vi "mathforthing.vi"(9 "setpoint":dbl, 10 "starting angle":dbl) -> (2 "output":dbl)   [LabVIEW 2020]
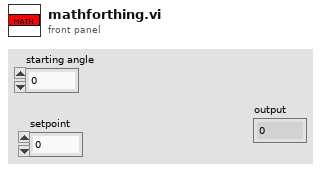
[diagram p1: front panel]
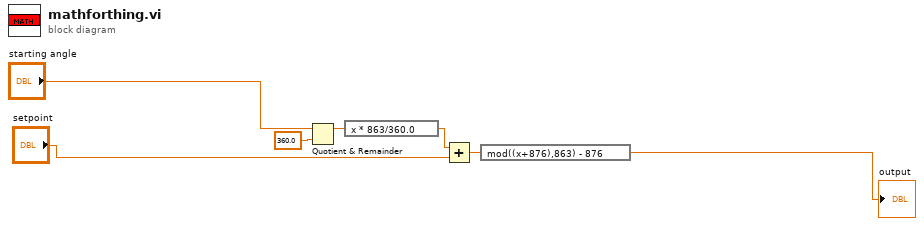
[diagram p0: block diagram]
diagram:
  n1 = Quotient & Remainder(x="starting angle", y=360.0) -> (x-y*floor(x/y)=w5:dbl)  [unwired: 1 out]
  n2 = expression code="x * 863/360.0"(w5) -> (w4:dbl)
  n3 = Add(x=w4, y="setpoint") -> (x+y=w7:dbl)
  n4 = expression code="mod((x+876),863) - 876"(w7) -> (→"output":dbl)
